vi "ENPH354_LabTracers.vi"() -> ()   [LabVIEW 2020]
uses:
  <vilib>/MakerHub/LINX/Public/Peripherals/Analog/Analog Read 1 Chan.vi
  <vilib>/MakerHub/LINX/Public/Peripherals/Analog/Analog Read N Chans.vi
  <vilib>/MakerHub/LINX/Private/Local IO/LinxAnalogRead.vi
  <vilib>/MakerHub/LINX/Public/Utilities/Check Channel.vi
  <vilib>/MakerHub/LINX/Public/Utilities/Open Serial.vi
  <vilib>/MakerHub/LINX/Private/Utilties/Generate Error.vi
  <vilib>/MakerHub/LINX/LMH-LINX.lvlib
panel:
  in  "Clear Graphs":bool
  in  "Save Point":bool
  out "LI":cluster{"X":dbl[], "Y":dbl[]}[](graph)
  out "LV":cluster{"X":dbl[], "Y":dbl[]}[](graph)
  out "IV":cluster{"X":dbl[], "Y":dbl[]}[](graph)
  out "Voltage":dbl(graph)
  out "error out":errorcluster
  in  "stop":bool
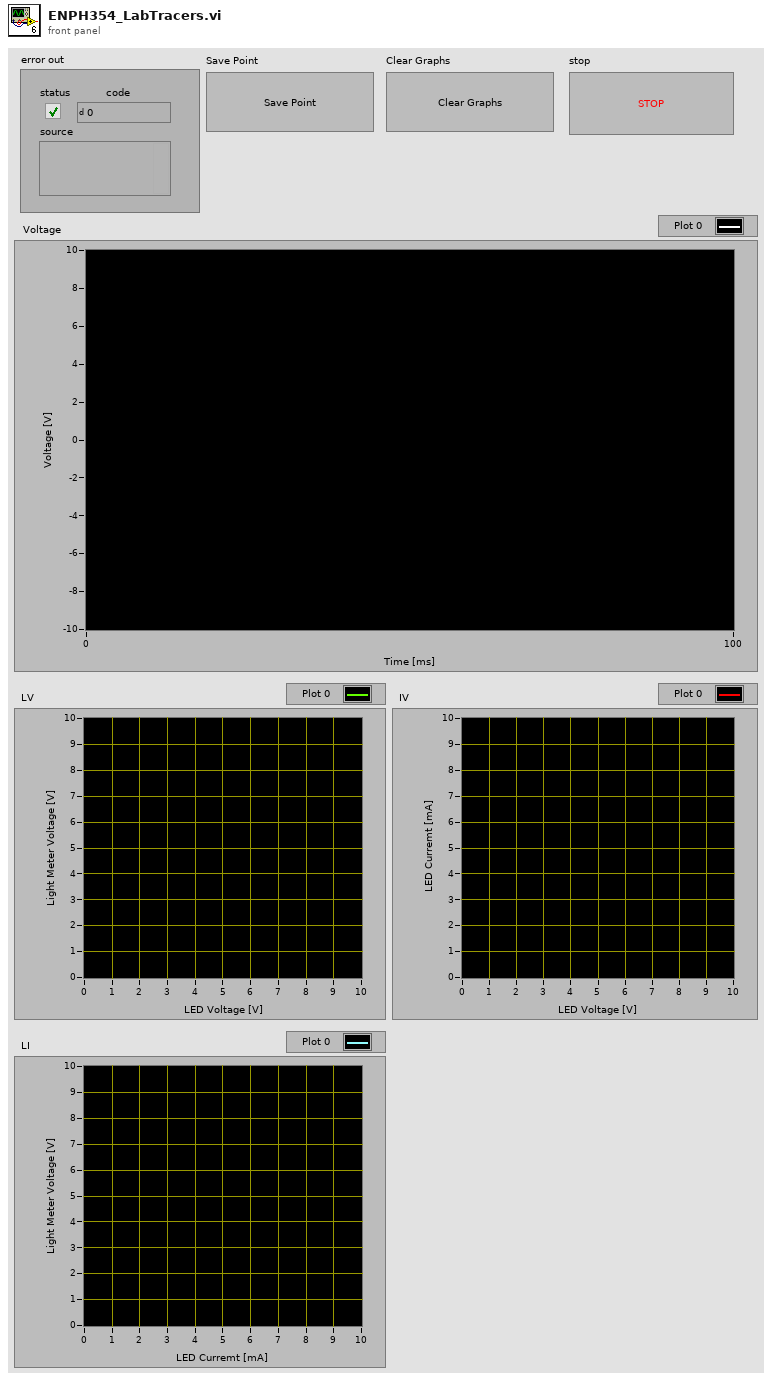
[diagram p1: front panel]
types:
  T1 = typedef "LMH-LINX.lvlib/LINX Ref.ctl" = cluster{"IO":T2, "Interface":T3, "LINX Device Config":T4}
  T2 = typedef "LMH-LINX.lvlib/Platform.ctl" = enum16{"Remote", "Local"}
  T3 = typedef "LMH-LINX.lvlib/Interface.ctl" = enum16{"Serial", "TCP"}
  T4 = typedef "LMH-LINX.lvlib/Device.lvlib/LINX Device Config.ctl" = cluster{"Interface":T3, "COM Port":refnum<visa-resource-name>, "TCP Configuration":T5, "Device Family":u8, "Device ID":u8, "Device Name":string, "TCP Ref":refnum<k5>, "Channels":T6}
  T5 = typedef "LMH-LINX.lvlib/Device.lvlib/TCP Config.ctl" = cluster{"IP Address":string, "Port":u16}
  T6 = typedef "LMH-LINX.lvlib/Channels.ctl" = cluster{"DI":u8[], "DO":u8[], "AI":u8[], "AO":u8[], "PWM":u8[], "QE":u8[], "UART":u8[], "I2C 2":u8[], "SPI":u8[], "CAN":u8[], "Servo":u8[], "AI Ref (V)":dbl, "AI Resolution (Bits)":u8, "AO Ref (V)":dbl, "AO Resolution (Bits)":u8}
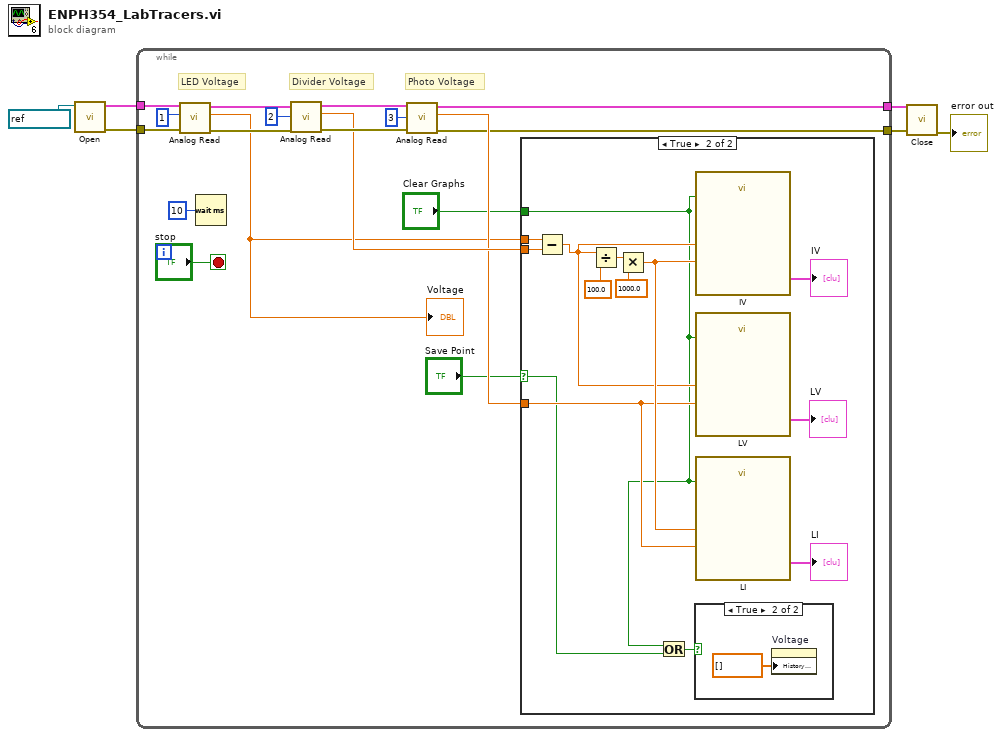
[diagram p0: block diagram]
diagram:
  n1 = call-poly <vilib>:"Open.vi"("Serial Port"=refnum<visa-resource-name> "COM7") -> ("Error Out"=w4:errorcluster, "LINX Resource"=w5:T1)  [unwired: 8 in, 1 out]
  n2 = while {
    tunnel: w5 -> [w22]
    tunnel: w4 -> [w21]
    tunnel: [w8] -> w2
    tunnel: [w7] -> w1
    stop <- "stop" stop-if-true
    # "Photo Voltage"
    # "Divider Voltage"
    # "LED Voltage"
    n3 = call-poly <vilib>:"Analog Read.vi"("Error In"=w21, "Analog Channel"=u8 1, "LINX Resource"=w22) -> ("Error Out"=w19:errorcluster, "Voltage"=w10:dbl, "LINX Resource"=w20:T1)  [unwired: 5 in, 1 out]
    "Voltage" <- w10
    n4 = Wait (ms)(milliseconds to wait=u32 10) -> ()  [unwired: 1 out]
    n5 = call-poly <vilib>:"Analog Read.vi"("Error In"=w19, "Analog Channel"=u8 2, "LINX Resource"=w20) -> ("Error Out"=w17:errorcluster, "Voltage"=w13:dbl, "LINX Resource"=w18:T1)  [unwired: 5 in, 1 out]
    n6 = call-poly <vilib>:"Analog Read.vi"("Error In"=w17, "Analog Channel"=u8 3, "LINX Resource"=w18) -> ("Error Out"=w7:errorcluster, "Voltage"=w12:dbl, "LINX Resource"=w8:T1)  [unwired: 5 in, 1 out]
    n7 = case shown="True" "Save Point" {
      selector: "Save Point" -> [_ w26]
      tunnel: w10 -> [_ w35]
      tunnel: w13 -> [_ w34]
      tunnel: w12 -> [_ w30]
      tunnel: "Clear Graphs" -> [_ w25]
      frame False {
      }
      frame True {
        n8 = Subtract(x=w35, y=w34) -> (x-y=w28:dbl)
        n9 = Divide(x=w28, y=100.0) -> (x/y=w33:dbl)
        n10 = Multiply(x=w33, y=1000.0) -> (x*y=w32:dbl)
        n11 = Or(x=w25, y=w26) -> (x .or. y?=w27:bool)
        n12 = case shown="True" w27 {
          frame False {
          }
          frame True {
            n13 = property on="Voltage" class="WFChart (strict)"("History Data"=dbl[] []) -> ()  [unwired: 2 in, 2 out]
          }
        }
        n14 = call "IV"("Reset"=w25, "Y Input"=w32, "X Input"=w28) -> ("XY Graph"=→"IV":cluster{"X":dbl[], "Y":dbl[]}[])  [unwired: 7 in, 1 out]
        n15 = call "LV"("Reset"=w25, "Y Input"=w30, "X Input"=w28) -> ("XY Graph"=→"LV":cluster{"X":dbl[], "Y":dbl[]}[])  [unwired: 7 in, 1 out]
        n16 = call "LI"("Reset"=w25, "Y Input"=w30, "X Input"=w32) -> ("XY Graph"=→"LI":cluster{"X":dbl[], "Y":dbl[]}[])  [unwired: 7 in, 1 out]
      }
    }
  }
  n17 = call <vilib>:"Close.vi"("Error In"=w1, "LINX Resource"=w2) -> ("Error Out"=→"error out":errorcluster)  [unwired: 9 in]
